vi "Add.vi"(8 "error in (no error)":errorcluster, 9 "Time (s)":dbl, 10 "Repetitions":u32, 11 "Error Code":i32) -> (0 "error out":errorcluster)   [LabVIEW 2026, in "TALOS.lvlib" / "Classes.lvlib" / "Error Filter.lvclass"]
doc: "Use this VI to add an error to be skipped in the future. If repetitions and time are both left to zero, the error will be permanently skipped: otherwise the error will be skipped until at least one of the two conditions will be met."
uses:
  Error Filter.lvclass
  Ancestor/Ancestor/Ancestor.lvclass/Ancestor.ctl
  Support VIs/Generate Error.vi
  FGV/Error Memory/Get Error Description.vi
  Support VIs/Get PC name.vi
  Ancestor/Ancestor/Read ID.vi
  Support VIs/Get Class Name.vi
  <vilib>/Utility/error.llb/Clear Errors.vi
  FGV/Error Memory/Error Memory Core.vi
  <vilib>/AdvancedString/Delimited String to 1D String Array.vi
  <vilib>/AdvancedString/Delimited String to 1D String Array (string).vi
  Support VIs/Circus Root Path.vi
  FGV/Error Memory/Error Crt Lvl checker.vi
  FGV/Error Memory/Error Memory Core.vi/40c8088d-b597-4017-91af-faa98e00292e.vi
  FGV/Error Memory/Error Memory Core.vi/d4a3ab98-063c-4e44-b43d-fbdcfe6c2be2.vi
  Support VIs/Global Memory.vi
  <vilib>/Utility/LVClass/Get LV Class Name.vi
  Support VIs/Is in Packed Library.vi
  Support VIs/TALOS Root path.vi
  Support VIs/Read CSV worksheet.vi
  Support VIs/Global Constants.vi
  <vilib>/Utility/error.llb/General Error Handler.vi
  Support VIs/Error Log.vi
  Ancestor/Ancestor/Ancestor.lvclass
  <vilib>/Comparison/Equal/Equal Functor/Equal Functor.lvclass
  TALOS.lvlib
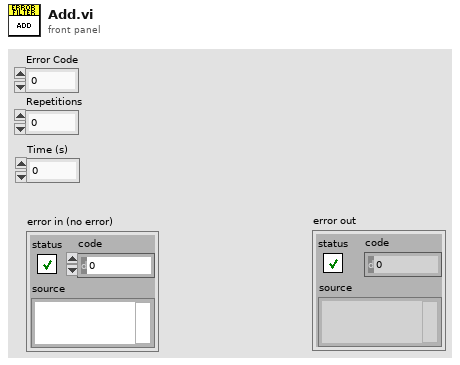
[diagram p1: front panel]
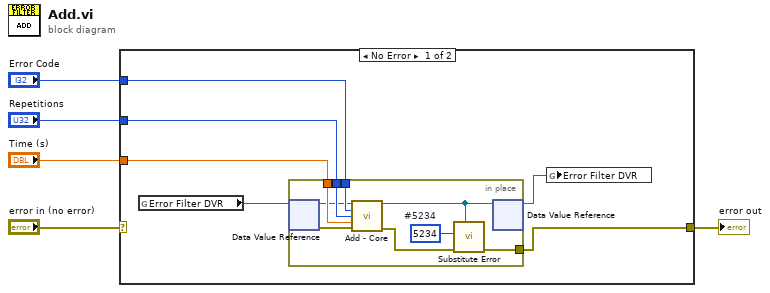
[diagram p0: block diagram]
diagram:
  n1 = case shown="No Error" "error in (no error)" {
    selector: "error in (no error)" -> [_ w21]
    tunnel: [w6 w21] -> w1
    tunnel: "Error Code" -> [w10 _]
    tunnel: "Repetitions" -> [w9 _]
    tunnel: "Time (s)" -> [w8 _]
    frame No Error {
      n2 = global read "Global Memory.vi" "Error Filter DVR"() -> (w11:refnum<data-value>)
      n3 = in-place {
        in-place-border: [w13] -> w6
        in-place-border: w10 -> [w20]
        in-place-border: w9 -> [w19]
        in-place-border: w8 -> [w18]
        w15 = 5234  # #5234
        n4 = in-place-dvr #1(w11) -> (w17:refnum<class "Error Filter.lvclass">, w16:errorcluster)
        n5 = call "Add - Core.vi"("Error Filter in"=w17, "Error Code"=w20, "Repetitions"=w19, "Time (s)"=w18, "error in (no error)"=w16) -> ("Error Filter out"=w12:refnum<class "Error Filter.lvclass">, "error out"=w14:errorcluster)  [unwired: 9 in]
        n6 = call "Substitute Error.vi"("LabVIEW Object"=w12, "error in (no error)"=w14, "Error Code"=w15) -> ("error out"=w13:errorcluster)  [unwired: 8 in]
        n7 = in-place-dvr #1(w12) -> (w7:refnum<data-value>)  [unwired: 1 out]
      }
      n8 = global write "Global Memory.vi" "Error Filter DVR"(w7) -> ()
    }
    frame Error {
    }
  }
  "error out" <- w1
